vi "PWM Output Post Step Type.vi"(8 "error in (no error)":errorcluster, 9 "PWM Output In":T1, 10 "Socket No":u16=1, 11 "NI PWM Output in":refnum<class "NI PWM Output.lvclass">) -> (0 "error out":errorcluster, 3 "NI PWM Output out":refnum<class "NI PWM Output.lvclass">)   [LabVIEW 2023, in "HardwareAbstractionLayer_LVOOP.lvlib" / "NI PWM Output.lvclass"]
uses:
  NI PWM Output.lvclass
  Control/PWM Output Edit.ctl
  NI PWM Output.lvclass/NI PWM Output.ctl
  Database/Database.lvclass
  <resource>/objmgr/daqmx.rc
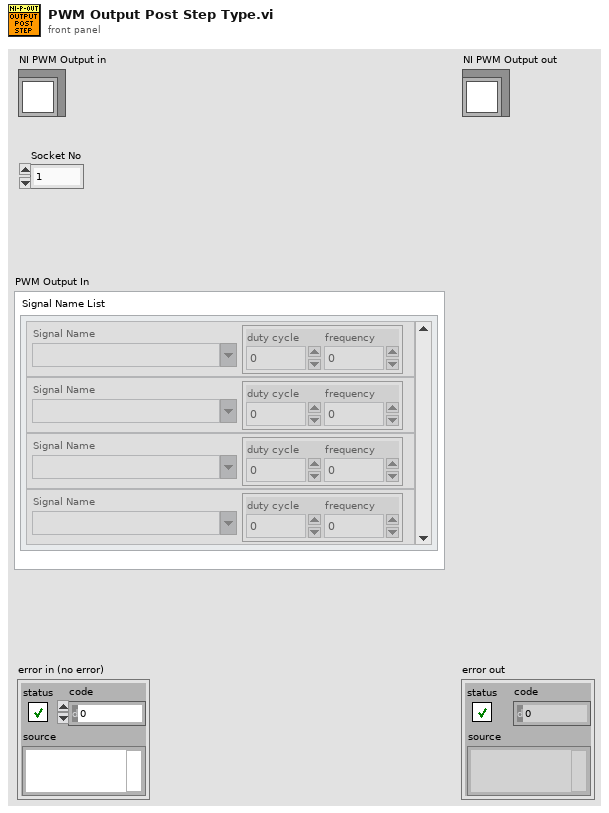
[diagram p1: front panel]
types:
  T1 = typedef "HardwareAbstractionLayer_LVOOP.lvlib/NI PWM Output.lvclass/PWM Output Edit.ctl" = cluster{"Signal Name List":cluster{"Signal Name":string, "values":cluster{"duty cycle":dbl, "frequency":dbl}}[]}
  T2 = cluster{"table":string, "condition":string, "columns":string[]}
  T3 = cluster{"Signal Name":string, "values":cluster{"duty cycle":dbl, "frequency":dbl}}[]
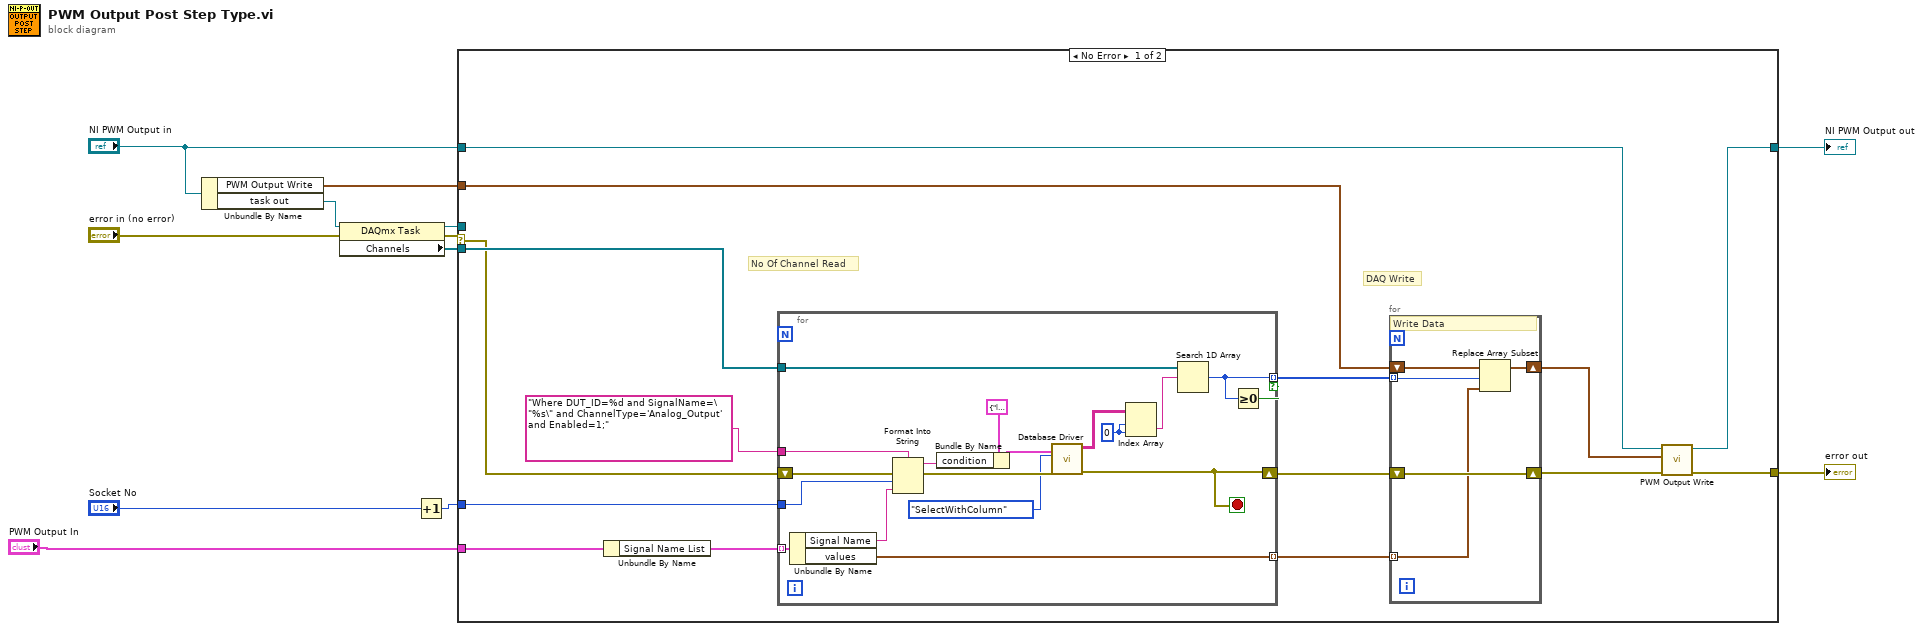
[diagram p0: block diagram]
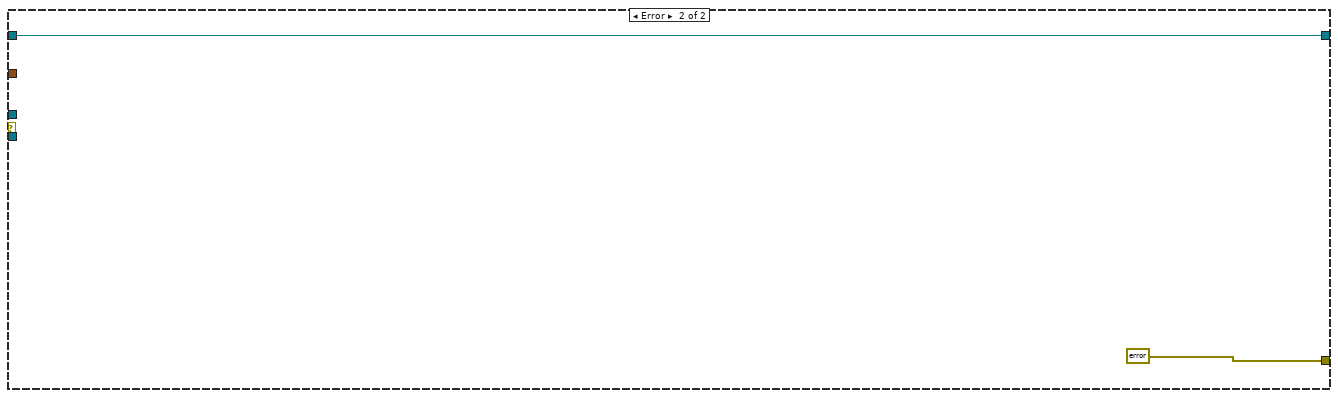
[diagram p2: hidden frame]
diagram:
  n1 = Unbundle By Name("NI PWM Output in") -> ("PWM Output Write"=w5:cluster{"duty cycle":dbl, "frequency":dbl}[], "task out"=w12:refnum<k21>)
  n2 = property class="DAQmx Task"(reference=w12, error in="error in (no error)") -> (reference out=w9:refnum<k21>, error out=w6:errorcluster, "Channels"=w8:refnum<k21>[])
  n3 = Increment(x="Socket No") -> (x+1=w10:u16)
  n4 = case shown="No Error" w6 {
    selector: w6 -> [w20 _]
    tunnel: [w14 errorcluster {"status"=TRUE, "code"=0, "source"="AO Task is not been created. please check in database."} ("error constant")] -> w2
    tunnel: "PWM Output In" -> [w24 _]
    tunnel: w9 -> [_ _]
    tunnel: w8 -> [w22 _]
    tunnel: w10 -> [w21 _]
    tunnel: w5 -> [w18 _]
    tunnel: "NI PWM Output in" -> [w17 w51]
    tunnel: [w13 w51] -> w3
    frame No Error {
      # "No Of Channel Read"
      # "DAQ Write"
      n5 = Unbundle By Name(w24) -> ("Signal Name List"=w27:T3)
      n6 = for {
        tunnel: w27 -> [w31] mode=indexing
        tunnel: "Where DUT_ID=%d and SignalName=\"%s\" and ChannelType='Analog_Output' and Enabled=1;" -> [w45]
        shift-right: [w33] -> w19
        shift-left: w20 -> [w41]
        tunnel: w22 -> [w38]
        tunnel: [w35] -> w25 mode=indexing if=w34
        tunnel: w21 -> [w32]
        tunnel: [w29] -> w23 mode=indexing
        stop <- w33 stop-if-true
        w37 = 0 ("disabled index (col)")
        n7 = Unbundle By Name(w31) -> ("Signal Name"=w30:string, "values"=w29:cluster{"duty cycle":dbl, "frequency":dbl})
        n8 = Format Into String(format string=w45, error in=w41, w32, w30) -> (resulting string=w43:string, error out=w40:errorcluster)  [unwired: 1 in]
        n9 = Bundle By Name(cluster=T2 {"table"="ltt.daq_configuration", "condition"="Where ChannelType='Analog_Input' and Enabled=1", "columns"=["PhysicalChannel"]} ("SQLTableData"), "condition"=w43) -> (w42:T2)
        n10 = call "Database Driver.vi"("SQLTableData"=w42, "error in"=w40, "Select"=enum16{"SelectWithQuery", "SelectWithColumn"}."SelectWithColumn") -> ("error out"=w33:errorcluster, "data"=w39:string[][])  [unwired: 5 in, 2 out]
        n11 = Index Array(array=w39, index (row)=w37, index (col)=w37) -> (element=w36:string)
        n12 = Search 1D Array(1D array=w38, element=w36) -> (index of element=w35:i32)  [unwired: 1 in]
        n13 = Greater Or Equal To 0?(x=w35) -> (x >= 0?=w34:bool)
      }
      n14 = for {
        shift-right: [w50] -> w16
        shift-left: w19 -> [w50]
        tunnel: w25 -> [w49] mode=indexing
        tunnel: w23 -> [w47] mode=indexing
        shift-right: [w46] -> w15
        shift-left: w18 -> [w48]
        # "Write Data"
        n15 = Replace Array Subset(array=w48, new element=w47, index=w49) -> (w46:cluster{"duty cycle":dbl, "frequency":dbl}[])
      }
      n16 = call-dynamic "PWM Output Write.vi"("error in"=w16, "PWM Output Write"=w15, "NI PWM Output in"=w17) -> ("error out"=w14:errorcluster, "NI PWM Output out"=w13:refnum<class "NI PWM Output.lvclass">)  [unwired: 7 in]
    }
    frame Error {
    }
  }
  "error out" <- w2
  "NI PWM Output out" <- w3
